vi "Acquire.vi"(8 "error in (no error)":errorcluster, 11 "Panel Control Counter in":refnum<class "Panel Control Counter.lvclass">) -> (0 "error out":errorcluster, 3 "Panel Control Counter out":refnum<class "Panel Control Counter.lvclass">)   [LabVIEW 2017, in "MGI-Panel Manager.lvlib" / "Panel Control Counter.lvclass"]
doc: "Acquires a Panel Control Counter.\n\n----\nPlease see the following web address for additional documentation and tutorial information:\nhttp://www.mooregoodideas.com/mgi-panel-manager/\n\nAuthor: Derek Trepanier\n\nCopyright (c) 2018, Moore Good Ideas, Inc.\n\nAll rights reserved.\n\nRedistribution and use in source and binary forms, with or without modification, are permitted provided that the following conditions are met:\n\n * Redistributions of source code must retain the above copyright notice, this list of conditions and the following disclaimer.\n * Redistributions in binary form must reproduce the above copyright notice, this list of conditions and the following disclaimer in the documentation and/or other materials provided with the distribution.\n * Neither the name of Moore Good Ideas, Inc. nor the names of its contributors may be used to endorse or promote products derived from this software without specific prior written permission.\n\nTHIS SOFTWARE IS PROVIDED BY THE COPYRIGHT HOLDERS AND CONTRIBUTORS \"AS IS\" AND ANY EXPRESS OR IMPLIED WARRANTIES, INCLUDING, BUT NOT LIMITED TO, THE IMPLIED WARRANTIES OF MERCHANTABILITY AND FITNESS FOR A PARTICULAR PURPOSE ARE DISCLAIMED. IN NO EVENT SHALL THE COPYRIGHT OWNER OR CONTRIBUTORS BE LIABLE FOR ANY DIRECT, INDIRECT, INCIDENTAL, SPECIAL, EXEMPLARY, OR CONSEQUENTIAL DAMAGES (INCLUDING, BUT NOT LIMITED TO, PROCUREMENT OF SUBSTITUTE GOODS OR SERVICES; LOSS OF USE, DATA, OR PROFITS; OR BUSINESS INTERRUPTION) HOWEVER CAUSED AND ON ANY THEORY OF LIABILITY, WHETHER IN CONTRACT, STRICT LIABILITY, OR TORT (INCLUDING NEGLIGENCE OR OTHERWISE) ARISING IN ANY WAY OUT OF THE USE OF THIS SOFTWARE, EVEN IF ADVISED OF THE POSSIBILITY OF SUCH DAMAGE."
uses:
  Panel Control Counter.lvclass
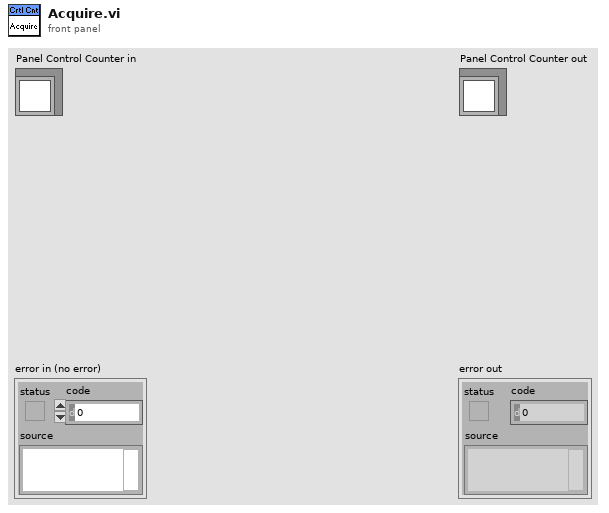
[diagram p1: front panel]
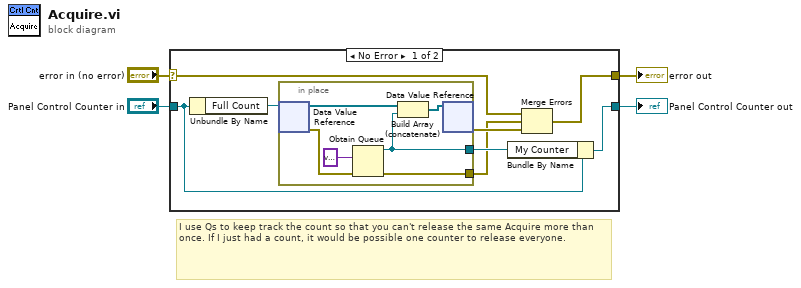
[diagram p0: block diagram]
diagram:
  # "I use Qs to keep track the count so that you can't release the same Acquire more than once. If I just had a count, it would be possible one counter to release everyone."
  n1 = case shown="No Error" "error in (no error)" {
    selector: "error in (no error)" -> [w11 w20]
    tunnel: [w9 w20] -> w3
    tunnel: "Panel Control Counter in" -> [w8 w19]
    tunnel: [w7 w19] -> w1
    frame No Error {
      n2 = Unbundle By Name(w8) -> ("Full Count"=w12:refnum<data-value>)
      n3 = in-place {
        in-place-border: [w15] -> w6
        in-place-border: [w13] -> w5
        n4 = in-place-dvr #1(w12) -> (w18:refnum<queue>[], w14:errorcluster)
        n5 = Obtain Queue(element data type=variant, error in (no error)=w14) -> (queue out=w15:refnum<queue>, error out=w13:errorcluster)  [unwired: 3 in, 1 out]
        n6 = Build Array (concatenate)(w18, w15) -> (w16:refnum<queue>[])
        n7 = in-place-dvr #1(w16) -> (w10:errorcluster)  [unwired: 1 out]
      }
      n8 = Bundle By Name(cluster=w8, "My Counter"=w6) -> (w7:refnum<class "Panel Control Counter.lvclass">)
      n9 = Merge Errors(w11, w5, w10) -> (w9:errorcluster)
    }
    frame Error {
    }
  }
  "error out" <- w3
  "Panel Control Counter out" <- w1
